vi "arduino_5_0.vi"() -> ()   [LabVIEW 2015]
uses:
  <vilib>/LabVIEW Interface for Arduino/LabVIEW Interface for Arduino.lvlib
panel:
  in  "constant value given by this instrument":dbl(slide) scale=0.0..180.0
  out "Servo angle (Degrees)":u8(knob)=15 scale=0.0..360.0
  in  "stop":bool
  out "IR range define":dbl(knob) scale=0.0..5.0
  in  "Analog Input Pin (0)":u8
  in  "DIO Pin (2)":u8=2
  in  "Servo Number (0)":u8
  in  "Number Of Servos (1)":u8=1
  in  "VISA resource":refnum<visa-resource-name>
  # "Servo project"
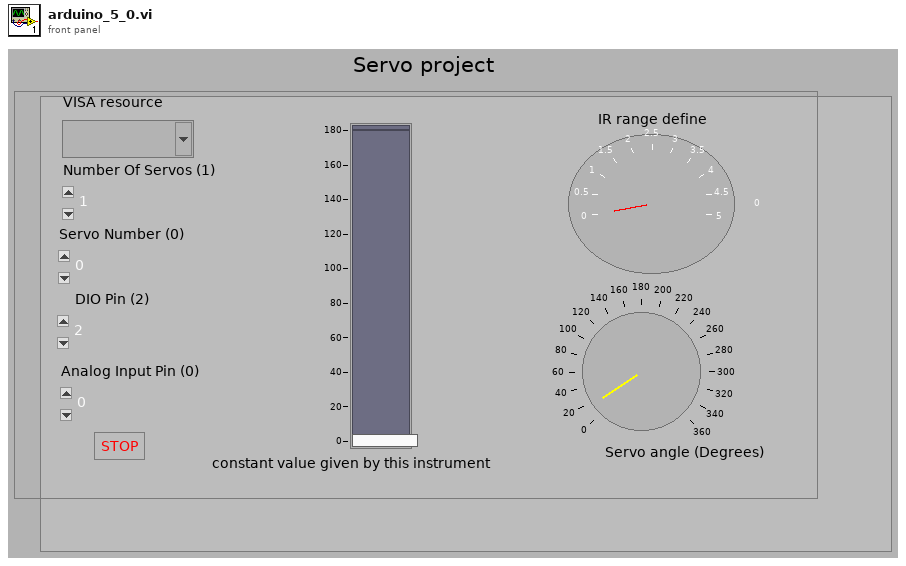
[diagram p1: front panel]
types:
  T1 = typedef "LabVIEW Interface for Arduino.lvlib/Arduino Resource.ctl" = cluster{"VISA resource":refnum<visa-resource-name>, "Board Type":T2, "Connection Type":enum8{"USB / Serial"}, "Bytes Per Packet (15)":u8}
  T2 = typedef "LabVIEW Interface for Arduino.lvlib/Board Type.ctl" = enum16{"Uno", "Dimuelanove w/Atmega 328", "Mega 2560"}
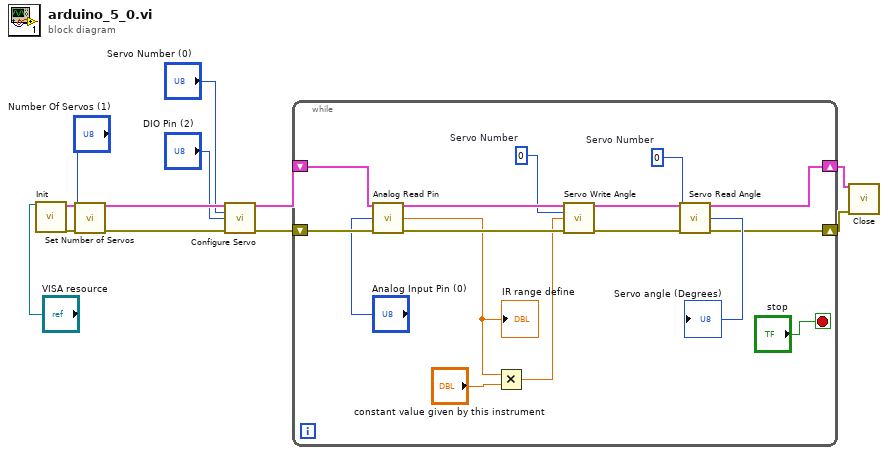
[diagram p0: block diagram]
diagram:
  n1 = call <vilib>:"Init.vi"("VISA resource"="VISA resource") -> ("Arduino Resource"=w12:T1, "error out"=w11:errorcluster)  [unwired: 17 in]
  n2 = call <vilib>:"Set Number of Servos.vi"("Arduino Resource"=w12, "Number Of Servos (1)"="Number Of Servos (1)", "error in"=w11) -> ("Arduino Resource"=w10:T1, "error out"=w9:errorcluster)  [unwired: 11 in]
  n3 = call <vilib>:"Configure Servo.vi"("Arduino Resource"=w10, "Servo Number (0)"="Servo Number (0)", "DIO Pin (2)"="DIO Pin (2)", "error in"=w9) -> ("Arduino Resource"=w8:T1, "error out"=w7:errorcluster)  [unwired: 10 in]
  n4 = while {
    shift-right: [w14] -> w2
    shift-left: w8 -> [w28]
    shift-right: [w13] -> w1
    shift-left: w7 -> [w25]
    stop <- "stop" stop-if-true
    w18 = u8 0  # Servo Number
    w21 = u8 0  # Servo Number
    n5 = call <vilib>:"Analog Read Pin.vi"("Arduino Resource"=w28, "Analog Input Pin (0)"="Analog Input Pin (0)", "error in"=w25) -> ("Arduino Resource"=w27:T1, "Voltage"=w20:dbl, "error out"=w24:errorcluster)  [unwired: 10 in]
    "IR range define" <- w20
    n6 = Multiply(x=w20, y="constant value given by this instrument") -> (x*y=w19:dbl)
    n7 = call <vilib>:"Servo Write Angle.vi"("Arduino Resource"=w27, "Servo Number"=w21, "Angle (Degrees)"=w19, "error in"=w24) -> ("Arduino Resource"=w26:T1, "error out"=w23:errorcluster)  [unwired: 10 in]
    n8 = call <vilib>:"Servo Read Angle.vi"("Arduino Resource"=w26, "Servo Number"=w18, "error in"=w23) -> ("Arduino Resource"=w14:T1, "Angle (Degrees)"=→"Servo angle (Degrees)":u8, "error out"=w13:errorcluster)  [unwired: 10 in]
  }
  n9 = call <vilib>:"Close.vi"("Arduino Resource"=w2, "error in"=w1) -> ()  [unwired: 13 in, 1 out]
